vi "Current Position.vi"(8 "error in (no error)":errorcluster, 11 "FHPP in":refnum<class "FHPP.lvclass">) -> (0 "error out":errorcluster, 1 "Vel (%)":u8, 2 "Position":u32, 3 "FHPP out":refnum<class "FHPP.lvclass">)   [LabVIEW 2022 SP3, in "FHPP.lvclass"]
uses:
  FHPP.lvclass
  FHPP.lvclass/FHPP.ctl
  TypeDefs/Operating Mode.ctl
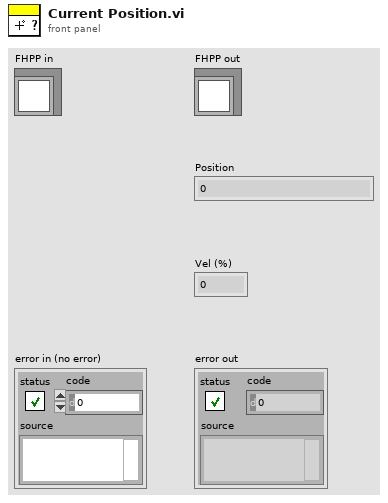
[diagram p1: front panel]
types:
  T1 = typedef "FHPP.lvclass/Operating Mode.ctl" = enum16{"Record Selection", "Direct Mode", "Reserved 1", "Reserved 2"}
  T2 = typedef "FHPP.lvclass/Setpoints.ctl" = cluster{"Vel/VelRamp (%)":u8, "Setpoint":u32}
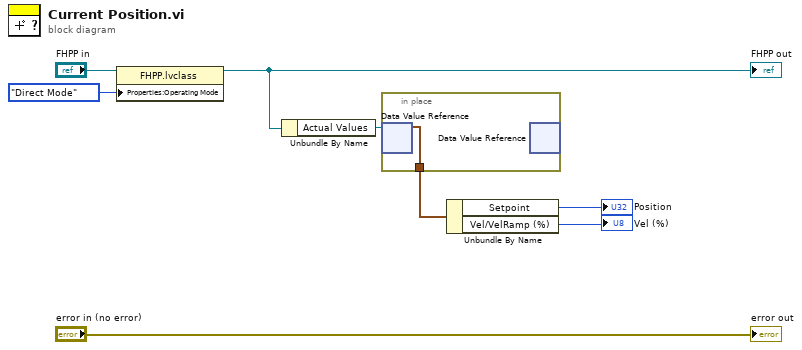
[diagram p0: block diagram]
diagram:
  n1 = property class="FHPP.lvclass"(reference="FHPP in", "Properties:Operating Mode"=Operating_Mode."Direct Mode" ("Operating Mode")) -> (reference out=w2:refnum<class "FHPP.lvclass">)  [unwired: 1 in, 1 out]
  "FHPP out" <- w2
  n2 = Unbundle By Name(w2) -> ("Actual Values"=w6:refnum<data-value>)
  n3 = in-place {
    in-place-border: [w9] -> w5
    n4 = in-place-dvr #1(w6) -> (w9:T2)  [unwired: 1 out]
    n5 = in-place-dvr #1() -> ()  [unwired: 1 in, 2 out]
  }
  n6 = Unbundle By Name(w5) -> ("Setpoint"=→"Position":u32, "Vel/VelRamp (%)"=→"Vel (%)":u8)
  "error out" <- "error in (no error)"
